vi "Detect Sign Change.vi"(1 "Input":dbl) -> (0 "Sign Changed?":bool)   [LabVIEW 2016]
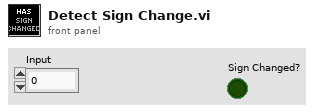
[diagram p1: front panel]
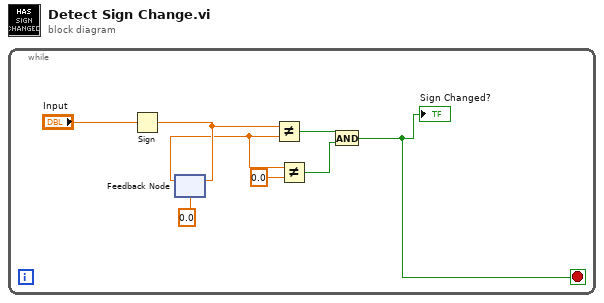
[diagram p0: block diagram]
diagram:
  n1 = while {
    stop <- w1 stop-if-true
    n2 = Sign(1:"Input") -> (0:w7:dbl)
    n3 = feedback #1(0.0) -> (w4:dbl)
    n4 = feedback-in #1(w7) -> ()
    n5 = Not Equal?(x=w7, y=w4) -> (x != y?=w5:bool)
    n6 = Not Equal?(x=w4, y=0.0) -> (x != y?=w2:bool)
    n7 = And(x=w5, y=w2) -> (x .and. y?=w1:bool)
    "Sign Changed?" <- w1
  }
